vi "Emergency_stop_Command_subVI.vi"(0 "TCP connection ID IN":refnum<k5>, 1 "Active Low":u32 format="%x", 2 "Port":tag="Dev1/port0" caption="USB6008Port", 3 "Rate":dbl=100.0 caption="Sample Rate (in Hz)" format="%0.2f", 4 "dioHigh":u32=255 caption="Active High" format="%x", 5 "ERROR IN":errorcluster, 6 "Delay to reset e-stop":dbl=10000.0, 7 "Slope":i32(ring)=10280 caption="Raising/Falling" items=["Rising"=10280, "Falling"=10171], 8 "Trigger Source":tag="/Dev1/PFI0") -> (14 "TCP Connection \nID out":refnum<k5>, 16 "E-Stop output":string="Emergency stop occured.\nHence aborts all operation", 17 "Estop Test Result":picture, 19 "ERROR OUT":errorcluster)   [LabVIEW 2017]
uses:
  <vilib>/DAQmx/write.llb/DAQmx Write (Digital U32 1Chan 1Samp).vi
  <vilib>/DAQmx/create/channels.llb/DAQmx Create Channel (DO-Digital Output).vi
  <vilib>/DAQmx/configure/timing.llb/DAQmx Timing (Sample Clock).vi
  <vilib>/DAQmx/configure/trigger.llb/DAQmx Start Trigger (Digital Edge).vi
  <vilib>/DAQmx/miscellaneous.llb/DAQmx Fill In Error Info.vi
panel:
  # "EMERGENCY STOP"
  # "Additional info:\n1. USB6008 PO.0&PO.1: Dev1/port0/line0:1\n        Dev1: Device connected to test pc\n        port0: Port of USB6008\n        Line0:1: Selects PO.0 & PO.1 for communication\n\n2. Active Low and Active High\n         Active Low: 0 enables the e-stop \n         Active High: FF disables the e-stop\n 3. Digital Source\n         Default trigger source is PFI0"
  # "Active Low"
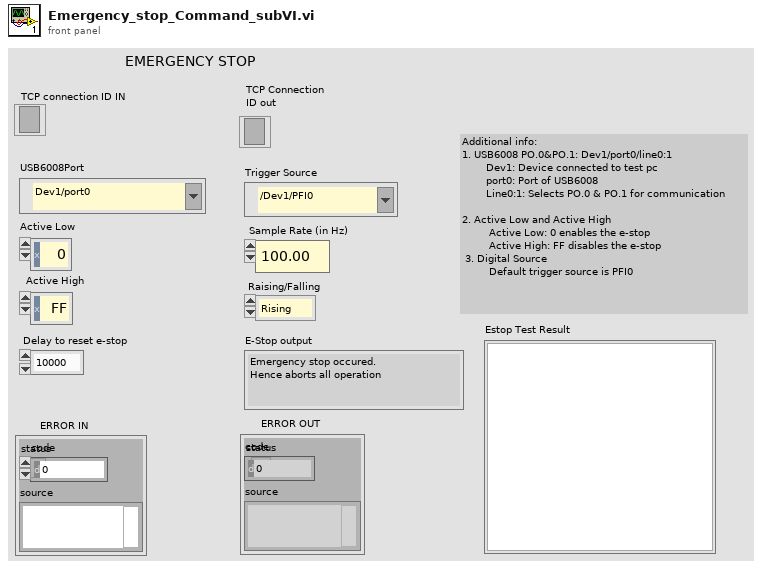
[diagram p1: front panel]
types:
  T1 = enum16{"Standard", "Buffered", "CRLF", "Immediate"}
  T2 = typedef "imagedata.ctl" = cluster{"image type":i32, "image depth":i32, "image":u8[], "mask":u8[], "colors":u32[], "Rectangle":cluster{"left":i16, "top":i16, "right":i16, "bottom":i16}}
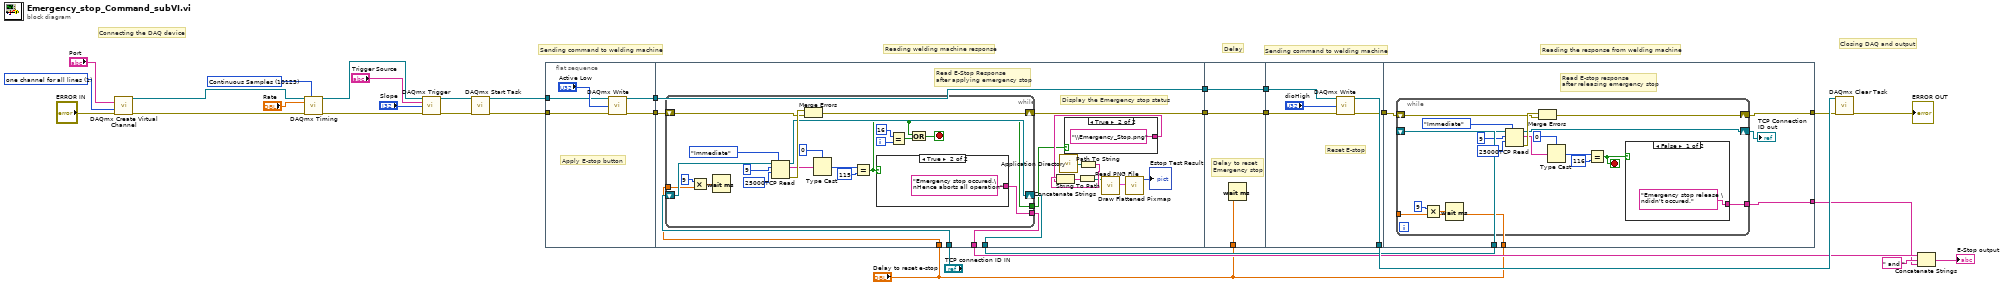
[diagram p0: block diagram]
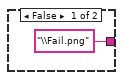
[diagram p2: hidden frame]
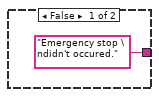
[diagram p3: hidden frame]
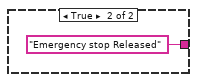
[diagram p4: hidden frame]
diagram:
  w29 = 10123 items=["Finite Samples"=10178, "Continuous Samples"=10123, "Hardware Timed Single Point"=12522] ("sample mode")
  w31 = 1 items=["one channel for each line", "one channel for all lines"] ("line grouping")
  # "Connecting the DAQ device"
  # "Closing DAQ and output"
  # "Reading the response from welding machine"
  # "Sending command to welding machine"
  # "Delay"
  # "Reading welding machine response"
  # "Sending command to welding machine"
  n1 = call-poly <vilib>:"DAQmx Create Virtual Channel.vi"("lines"="Port", "line grouping"=w31, "error in"="ERROR IN") -> ("task out"=w28:refnum<k21>, "error out"=w27:errorcluster)  [unwired: 11 in]
  n2 = call-poly <vilib>:"DAQmx Timing.vi"("task/channels in"=w28, "sample mode"=w29, "rate"="Rate", "error in"=w27) -> ("task out"=w24:refnum<k21>, "error out"=w25:errorcluster)  [unwired: 10 in]
  n3 = call-poly <vilib>:"DAQmx Trigger.vi"("task/channels in"=w24, "source"="Trigger Source", "edge"="Slope", "error in"=w25) -> ("task out"=w22:refnum<k21>, "error out"=w21:errorcluster)  [unwired: 10 in]
  n4 = call <vilib>:"DAQmx Start Task.vi"("task/channels in"=w22, "error in"=w21) -> ("task out"=w20:refnum<k21>, "error out"=w19:errorcluster)  [unwired: 12 in]
  n5 = flat-sequence {
    tunnel: w20 -> [w36]
    tunnel: w19 -> [w35]
    tunnel: [w34] -> w16
    tunnel: [w33] -> w14
    tunnel: w16 -> [w52]
    tunnel: [w51] -> w5
    tunnel: [w50] -> w3
    tunnel: w14 -> [w50]
    tunnel: "TCP connection ID IN" -> [w49]
    tunnel: "Delay to reset e-stop" -> [w48]
    tunnel: [w47] -> w12
    tunnel: [w46] -> w7
    tunnel: w5 -> [w80]
    tunnel: [w80] -> w4
    tunnel: w3 -> [w79]
    tunnel: [w79] -> w2
    tunnel: "Delay to reset e-stop" -> [w78]
    tunnel: [w85] -> w15
    tunnel: w4 -> [w84]
    tunnel: w2 -> [w82]
    tunnel: [w81] -> w11
    tunnel: w12 -> [w91]
    tunnel: w11 -> [w90]
    tunnel: [w89] -> w10
    tunnel: "Delay to reset e-stop" -> [w88]
    tunnel: [w87] -> w6
    frame #0 {
      # "Apply E-stop button"
      n6 = call-poly <vilib>:"DAQmx Write.vi"("task/channels in"=w36, "data"="Active Low", "error in"=w35) -> ("task out"=w33:refnum<k21>, "error out"=w34:errorcluster)  [unwired: 10 in, 1 out]
    }
    frame #1 {
      # "Display the Emergency stop status"
      # "Read E-Stop Response \nafter applying emergency stop"
      n7 = while {
        shift-right: [w71] -> w51
        shift-left: w52 -> [w74]
        shift-right: [w68] -> w47
        shift-left: w49 -> [w69]
        tunnel: w48 -> [w61]
        tunnel: [w60] -> w46
        tunnel: [w55] -> w38
        i -> [w59]
        stop <- w56 stop-if-true
        n8 = Multiply(x=9 ("bytes to read"), y=w61) -> (x*y=w62:dbl)
        n9 = Wait (ms)(milliseconds to wait=w62) -> ()  [unwired: 1 out]
        n10 = TCP Read(connection ID=w69, bytes to read=9, 7:T1."Immediate" ("mode (standard)"), 9:25000 ("timeout ms (25000)")) -> (connection ID out=w68:refnum<k5>, data out=w67:string, error out=w75:errorcluster)  [unwired: 1 in]
        n11 = Merge Errors(w75, w74) -> (w71:errorcluster)
        n12 = Type Cast(type=0 ("timeout ms (25000)"), x=w67) -> (*(type *) &x=w65:i32)
        n13 = Equal?(x=w65, y=115) -> (x = y?=w55:bool)
        n14 = case shown="True" w55 {
          tunnel: ["Emergency stop \ndidn't occured." "Emergency stop occured.\nHence aborts all operation"] -> w60
          frame False {
          }
          frame True {
          }
        }
        n15 = Equal?(x=16, y=w59) -> (x = y?=w57:bool)
        n16 = Or(x=w55, y=w57) -> (x .or. y?=w56:bool)
      }
      n17 = call <vilib>:"Application Directory.vi"() -> ("Application Directory"=w45:path)
      n18 = case shown="True" w38 {
        tunnel: ["\\Fail.png" ("string") "\\Emergency_Stop.png" ("string")] -> w39
        frame False {
        }
        frame True {
        }
      }
      n19 = Path To String(path=w45) -> (string=w44:string)
      n20 = Concatenate Strings(w44, w39) -> (w43:string)
      n21 = String To Path(string=w43) -> (path=w40:path)
      n22 = call <vilib>:"Read PNG File.vi"("path to PNG file"=w40) -> ("image data"=w42:T2)  [unwired: 8 in, 2 out]
      n23 = call <vilib>:"Draw Flattened Pixmap.vi"("image data"=w42) -> ("new picture"=→"Estop Test Result":picture)  [unwired: 8 in]
    }
    frame #2 {
      # "Delay to reset \nEmergency stop"
      n24 = Wait (ms)(milliseconds to wait=w78) -> ()  [unwired: 1 out]
    }
    frame #3 {
      # "Reset E-stop"
      n25 = call-poly <vilib>:"DAQmx Write.vi"("task/channels in"=w82, "data"="dioHigh", "error in"=w84) -> ("task out"=w85:refnum<k21>, "error out"=w81:errorcluster)  [unwired: 10 in, 1 out]
    }
    frame #4 {
      # "Read E-stop response\nafter releasing emergency stop"
      n26 = while {
        shift-right: [w104] -> w89
        shift-left: w90 -> [w107]
        shift-right: [w101] -> w86
        shift-left: w91 -> [w102]
        tunnel: w88 -> [w94]
        tunnel: [w92] -> w87
        stop <- w93 stop-if-true
        n27 = Multiply(x=9 ("bytes to read"), y=w94) -> (x*y=w95:dbl)
        n28 = Wait (ms)(milliseconds to wait=w95) -> ()  [unwired: 1 out]
        n29 = TCP Read(connection ID=w102, bytes to read=9, 7:T1."Immediate" ("mode (standard)"), 9:25000 ("timeout ms (25000)")) -> (connection ID out=w101:refnum<k5>, data out=w100:string, error out=w108:errorcluster)  [unwired: 1 in]
        n30 = Merge Errors(w108, w107) -> (w104:errorcluster)
        n31 = Type Cast(type=0 ("timeout ms (25000)"), x=w100) -> (*(type *) &x=w98:i32)
        n32 = Equal?(x=w98, y=116) -> (x = y?=w93:bool)
        n33 = case shown="False" w93 {
          tunnel: ["Emergency stop release \ndidn't occured." "Emergency stop Released"] -> w92
          frame False {
          }
          frame True {
          }
        }
      }
      "TCP Connection \nID out" <- w86
    }
  }
  n34 = call <vilib>:"DAQmx Clear Task.vi"("task in"=w15, "error in"=w10) -> ("error out"=→"ERROR OUT":errorcluster)  [unwired: 13 in]
  n35 = Concatenate Strings(w7, " and ", w6) -> (→"E-Stop output":string)
